vi "odor temporal control, no logging.vi"() -> ()   [LabVIEW 2013]
uses:
  <vilib>/DAQmx/write.llb/DAQmx Write (Digital Bool 1Line 1Point).vi
  Image Aquisition - Labview/Image Recorder/experiment state global.vi
  <vilib>/DAQmx/miscellaneous.llb/DAQmx Fill In Error Info.vi
panel:
  out "odor vs. time":waveform(dbl)(graph)={"t0"=timestamp(4109676248 s since 1904-01-01), "dt"=1.0, "Y"=[0.43491621316601353]}
  in  "direct control of digital lines":bool
  in  "digital controls":T1
  out "flow rates":T2={"air"=0.004776097601279616, "odor1"=10.169737786054611, "odor2"=1.3895910303108394, "co2"=13.005789695307612, "pid reading"=0.43491621316601353} {"pid reading" format="%0.2f"}
  out "setpoints":T3
  in  "gradient settings":T4={"air settings"={"enabled"=TRUE, "temporal ramp type"=enum."Square", "period(s)"=1200.0, "high limit"=1.0, "low limit"=1.0, "duty cycle (sq wave)"=50.0, "phase shift (deg)"=0.0, "value to output when disabled"=0.0}, "odor1 settings"={"enabled"=TRUE, "temporal ramp type"=enum."Sine", "period(s)"=120.0, "high limit"=50.0, "low limit"=0.0, "duty cycle (sq wave)"=50.0, "phase shift (deg)"=0.0, "value to output when disabled"=0.0}, "odor2 settings"={"enabled"=FALSE, "temporal ramp type"=enum."Sine", "period(s)"=120.0, "high limit"=100.0, "low limit"=0.0, "duty cycle (sq wave)"=50.0, "phase shift (deg)"=0.0, "value to output when disabled"=0.0}, "co2 settings"={"enabled"=FALSE, "temporal ramp type"=enum."Triangle", "period(s)"=200.0, "high limit"=200.0, "low limit"=0.0, "duty cycle (sq wave)"=50.0, "phase shift (deg)"=-90.0, "value to output when disabled"=0.0}} {"co2 settings"."value to output when disabled" min=0.0; "co2 settings"."low limit" format="%#_6p"; "odor2 settings"."value to output when disabled" max=100.0; "odor2 settings"."low limit" format="%#_6p"; "odor2 settings"."high limit" max=100.0; "odor1 settings"."value to output when disabled" max=100.0; "odor1 settings"."low limit" format="%#_6p"; "odor1 settings"."high limit" max=100.0; "air settings"."value to output when disabled" max=100.0; "air settings"."low limit" format="%#_6p"; "air settings"."high limit" max=100.0}
  in  "Sync Gradient To Image Aquisition":bool=TRUE
  in  "enable gradient":bool
  in  "restart gradient":bool
  in  "update period (ms)":u32=100
  in  "stop":bool
  out "error out":errorcluster
  # "restarting gradient also enables output"
  # "maximum amplitude is 100"
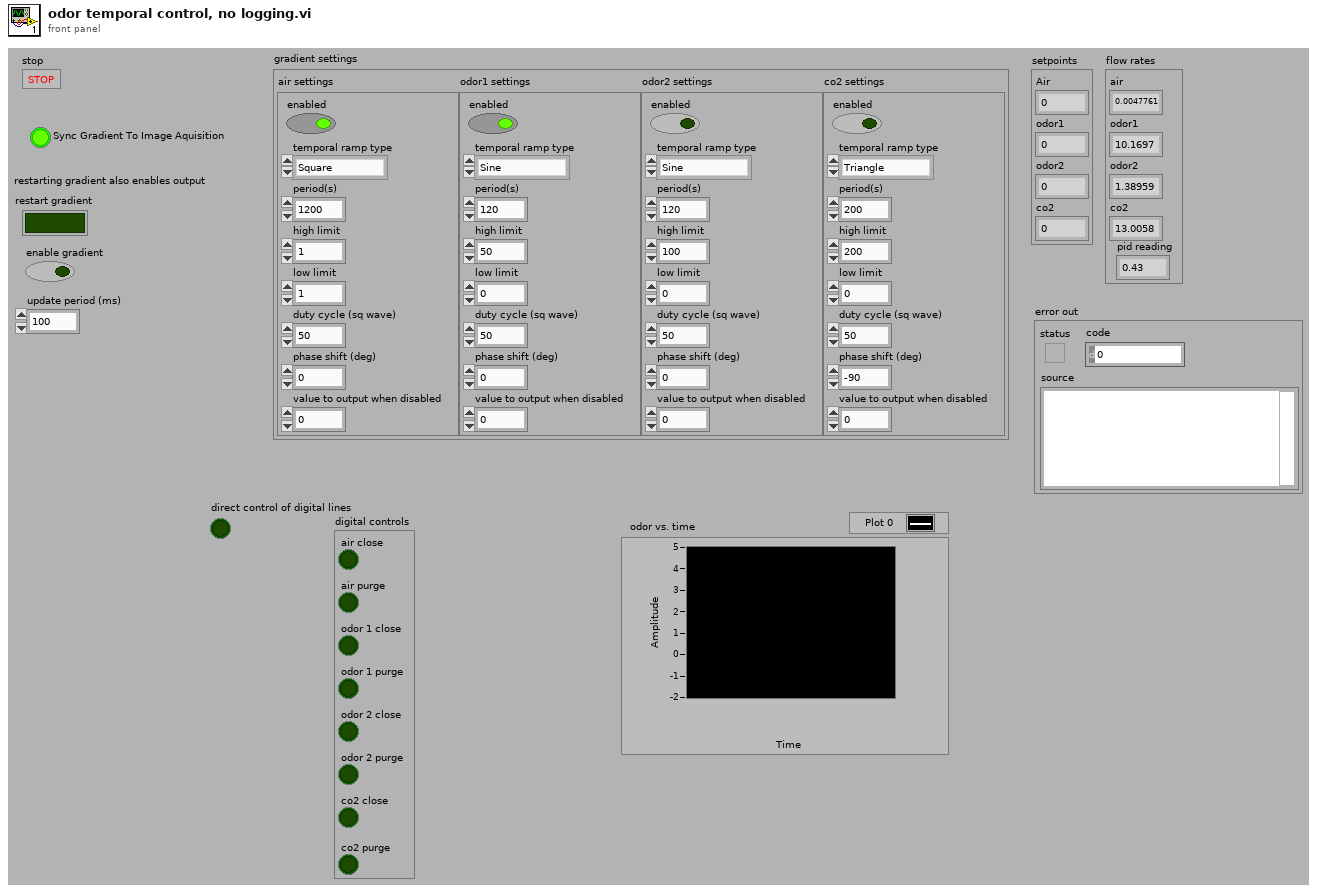
[diagram p1: front panel]
types:
  T1 = cluster{"air close":bool, "air purge":bool, "odor 1 close":bool, "odor 1 purge":bool, "odor 2 close":bool, "odor 2 purge":bool, "co2 close":bool, "co2 purge":bool}
  T2 = cluster{"air":dbl, "odor1":dbl, "odor2":dbl, "co2":dbl, "pid reading":dbl}
  T3 = cluster{"Air ":dbl, "odor1":dbl, "odor2":dbl, "co2":dbl}
  T4 = cluster{"air settings":cluster{"enabled":bool, "temporal ramp type":enum16{"Sine", "Triangle", "Sawtooth", "Square", "Exponential"}, "period(s)":dbl, "high limit":dbl, "low limit":dbl, "duty cycle (sq wave)":dbl, "phase shift (deg)":dbl, "value to output when disabled":dbl}, "odor1 settings":cluster{"enabled":bool, "temporal ramp type":enum16{"Sine", "Triangle", "Sawtooth", "Square", "Exponential"}, "period(s)":dbl, "high limit":dbl, "low limit":dbl, "duty cycle (sq wave)":dbl, "phase shift (deg)":dbl, "value to output when disabled":dbl}, "odor2 settings":cluster{"enabled":bool, "temporal ramp type":enum16{"Sine", "Triangle", "Sawtooth", "Square", "Exponential"}, "period(s)":dbl, "high limit":dbl, "low limit":dbl, "duty cycle (sq wave)":dbl, "phase shift (deg)":dbl, "value to output when disabled":dbl}, "co2 settings":cluster{"enabled":bool, "temporal ramp type":enum16{"Sine", "Triangle", "Sawtooth", "Square", "Exponential"}, "period(s)":dbl, "high limit":dbl, "low limit":dbl, "duty cycle (sq wave)":dbl, "phase shift (deg)":dbl, "value to output when disabled":dbl}}
  T5 = cluster{"analog output channels":cluster{"air ao":refnum<k21>, "odor 1 ao":refnum<k21>, "odor 2 ao":refnum<k21>, "co2 ao":refnum<k21>}, "analog input channels":cluster{"air ai":refnum<k21>, "odor 1 ai":refnum<k21>, "odor 2 ai":refnum<k21>, "co2 ai":refnum<k21>, "pid sensor 1 ai":refnum<k21>, "pid sensor 2 ai":refnum<k21>}, "digital control lines":cluster{"air close":refnum<k21>, "air purge":refnum<k21>, "odor 1 close":refnum<k21>, "odor 1 purge":refnum<k21>, "odor 2 close":refnum<k21>, "odor 2 purge":refnum<k21>, "co2 close":refnum<k21>, "co2 purge":refnum<k21>}}
  T6 = cluster{"experiment started":bool, "experiment ended":bool, "experiment start time":u32}
  T7 = cluster{"air close":refnum<k21>, "air purge":refnum<k21>, "odor 1 close":refnum<k21>, "odor 1 purge":refnum<k21>, "odor 2 close":refnum<k21>, "odor 2 purge":refnum<k21>, "co2 close":refnum<k21>, "co2 purge":refnum<k21>}
  T8 = cluster{"data directory":path, "file stub":string}
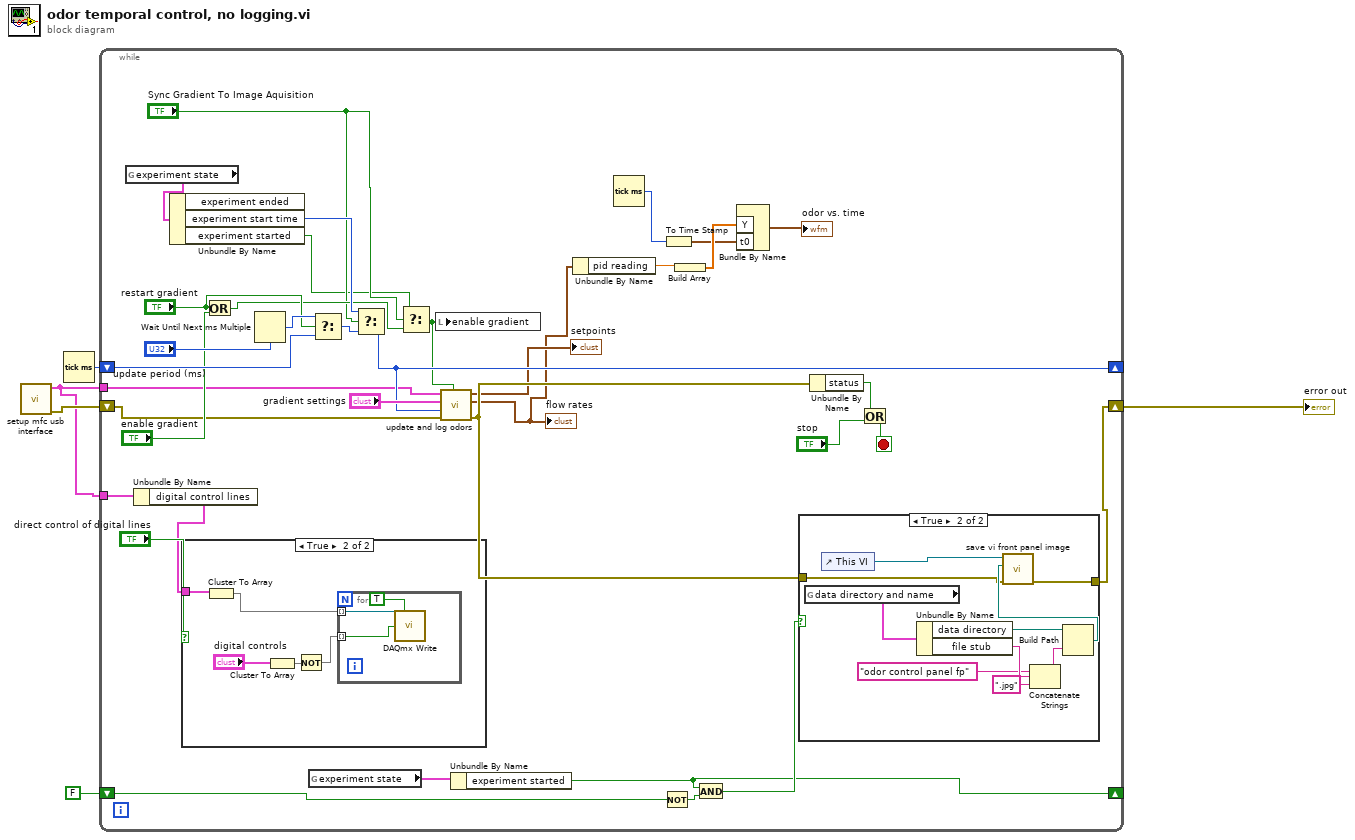
[diagram p0: block diagram]
diagram:
  n1 = call "setup mfc usb interface.vi"() -> ("error out"=w4:errorcluster, "daqmx tasks"=w1:T5)  [unwired: 10 in]
  n2 = Tick Count (ms)() -> (millisecond timer value=w5:u32)
  n3 = while {
    shift-right: [w22] -> w3
    shift-left: w4 -> [w19]
    shift-right: [w20] -> _
    shift-left: w5 -> [w38]
    tunnel: w1 -> [w17]
    shift-right: [w24] -> _
    shift-left: FALSE ("experiment started") -> [w23]
    tunnel: w1 -> [w14]
    stop <- w41 stop-if-true
    n4 = global read "experiment state global.vi" "experiment state"() -> (w33:T6)
    n5 = Unbundle By Name(w14) -> ("digital control lines"=w12:T7)
    n6 = Unbundle By Name(w33) -> ("experiment start time"=w32:u32, "experiment started"=w28:bool)  [unwired: 1 out]
    n7 = case shown="True" "direct control of digital lines" {
      tunnel: w12 -> [_ w45]
      frame False {
      }
      frame True {
        n8 = Cluster To Array(cluster=w45) -> (array=w43:refnum<k21>[])
        n9 = Cluster To Array(cluster="digital controls") -> (array=w44:bool[])
        n10 = Not(x=w44) -> (.not. x?=w42:bool[])
        n11 = for {
          tunnel: w43 -> [w49] mode=indexing
          tunnel: w42 -> [w48] mode=indexing
          n12 = call-poly <vilib>:"DAQmx Write.vi"("task/channels in"=w49, "auto start"=TRUE, "data"=w48) -> ()  [unwired: 10 in, 3 out]
        }
      }
    }
    n13 = Or(x="restart gradient", y="enable gradient") -> (x .or. y?=w31:bool)
    n14 = Wait Until Next ms Multiple(millisecond multiple="update period (ms)") -> (millisecond timer value=w37:u32)
    n15 = global read "experiment state global.vi" "experiment state"() -> (w25:T6)
    n16 = Select(t=w37, s="restart gradient", f=w38) -> (s? t:f=w34:u32)
    n17 = Select(t=w32, s="Sync Gradient To Image Aquisition", f=w34) -> (s? t:f=w20:u32)
    n18 = Select(t=w28, s="Sync Gradient To Image Aquisition", f=w31) -> (s? t:f=w18:bool)
    n19 = local write "enable gradient"(w18) -> ()
    n20 = call "update and log odors.vi"("global enable"=w18, "error in"=w19, "t0"=w20, "gradient settings"="gradient settings", "daqmx tasks"=w17) -> ("error out"=w16:errorcluster, "flow rates"=w11:T2, "setpoints"=→"setpoints":T3)  [unwired: 4 in]
    "flow rates" <- w11
    n21 = Unbundle By Name(w25) -> ("experiment started"=w24:bool)
    n22 = Unbundle By Name(w11) -> ("pid reading"=w10:dbl)
    n23 = Tick Count (ms)() -> (millisecond timer value=w7:u32)
    n24 = Not(x=w23) -> (.not. x?=w27:bool)
    n25 = To Time Stamp(1:w7) -> (0:w6:timestamp)
    n26 = Build Array(w10) -> (w9:dbl[])
    n27 = And(x=w24, y=w27) -> (x .and. y?=w26:bool)
    n28 = Bundle By Name("Y"=w9, "t0"=w6) -> (→"odor vs. time":waveform(dbl))  [unwired: 1 in]
    n29 = case shown="True" w26 {
      tunnel: [w50 w52] -> w22
      tunnel: w16 -> [w50 w51]
      frame False {
      }
      frame True {
        n30 = global read "experiment state global.vi" "data directory and name"() -> (w59:T8)
        n31 = control-ref of="This VI"() -> (w60:refnum<vi>)
        n32 = Unbundle By Name(w59) -> ("data directory"=w58:path, "file stub"=w57:string)
        n33 = Concatenate Strings("odor control panel fp" ("string"), w57, ".jpg" ("string")) -> (w54:string)
        n34 = Build Path(base path=w58, name or relative path=w54) -> (appended path=w53:path)
        n35 = call "save vi front panel image.vi"("error in (no error)"=w51, "path to JPEG file"=w53, "This VI"=w60) -> ("error out"=w52:errorcluster)  [unwired: 8 in]
      }
    }
    n36 = Unbundle By Name(w16) -> ("status"=w35:bool)
    n37 = Or(x=w35, y="stop") -> (x .or. y?=w41:bool)
  }
  "error out" <- w3
